vi "SHA-1 Core.vi"(0 "s1":u32=1732584193 format="%.0x", 1 "Input Bytes":u8[](array[numeric]), 5 "s2":u32=4023233417 format="%.0x", 7 "s3":u32=2562383102 format="%.0x", 9 "s4":u32=271733878 format="%.0x", 11 "s5":u32=271733878 format="%.0x") -> (4 "s1 out":u32, 6 "s2 out":u32, 8 "s3 out":u32, 10 "s4 out":u32, 15 "s5 out":u32)   [LabVIEW 2015, in "Front Panel Publisher.lvlib"]
doc: "This VI contains the core of the MD5 algorithm."
uses:
  Front Panel Publisher.lvlib
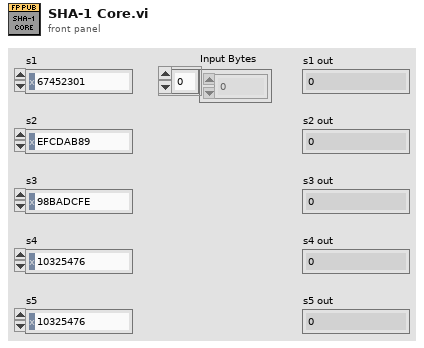
[diagram p1: front panel]
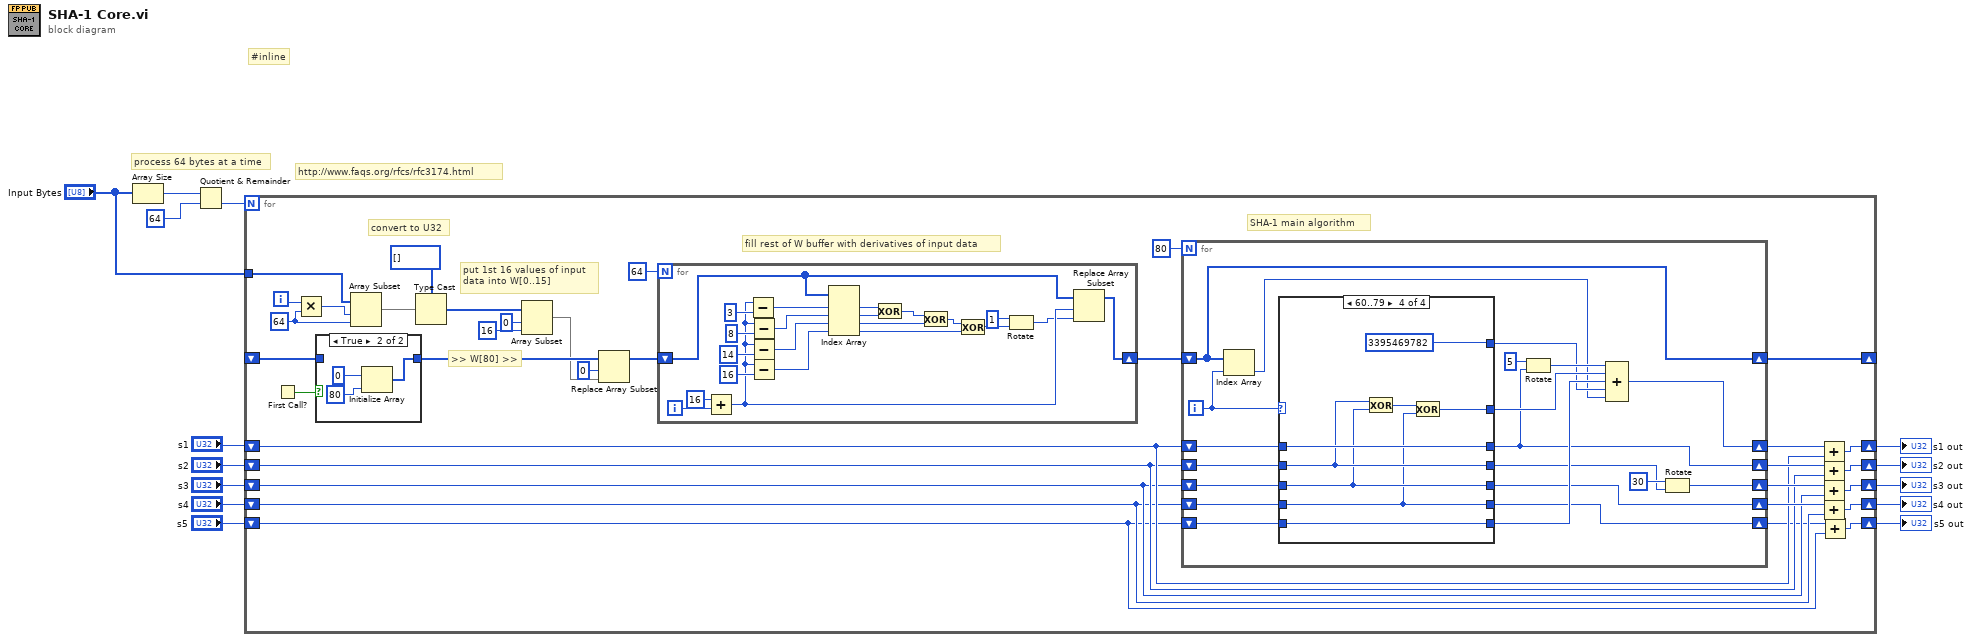
[diagram p0: block diagram]
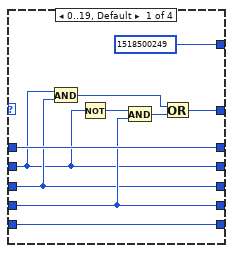
[diagram p2: hidden frame]
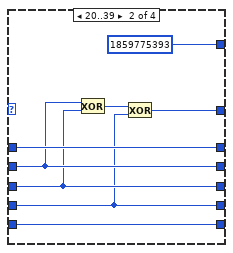
[diagram p3: hidden frame]
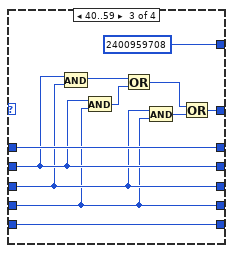
[diagram p4: hidden frame]
diagram:
  # "#inline"
  # "process 64 bytes at a time"
  # "http://www.faqs.org/rfcs/rfc3174.html"
  n1 = Array Size(array="Input Bytes") -> (size(s)=w2:i32)
  n2 = Quotient & Remainder(x=w2, y=64) -> (floor(x/y)=w14:i32)  [unwired: 1 out]
  n3 = for {
    N: w14 -> [_]
    shift-right: [w44] -> w12
    shift-left: "s1" -> [w40]
    shift-right: [w43] -> w11
    shift-left: "s2" -> [w39]
    shift-right: [w42] -> w10
    shift-left: "s3" -> [w38]
    shift-right: [w41] -> w9
    shift-left: "s4" -> [w37]
    tunnel: "Input Bytes" -> [w33]
    shift-right: [w34] -> w3
    shift-left: "s5" -> [w30]
    shift-right: [w19] -> _
    shift-left: _ -> [w24]
    i -> [w36]
    w32 = 64 ("y")
    # "SHA-1 main algorithm"
    # "fill rest of W buffer with derivatives of input data"
    # ">> W[80] >>"
    # "put 1st 16 values of input data into W[0..15]"
    # "convert to U32"
    n4 = First Call?() -> (First Call?: T/F=w26:bool)
    n5 = Multiply(x=w36, y=w32) -> (x*y=w31:i32)
    n6 = case shown="True" w26 {
      tunnel: [w128 w130] -> w25
      tunnel: w24 -> [w128 _]
      frame False {
      }
      frame True {
        n7 = Initialize Array(u32 0 ("y"), 80 ("dimension size")) -> (w130:u32[])
      }
    }
    n8 = Array Subset(array=w33, index=w31, length=w32) -> (w28:u8[])
    n9 = Type Cast(type=u32[] [], x=w28) -> (*(type *) &x=w27:u32[])
    n10 = Array Subset(array=w27, index=0, length=16) -> (w18:u32[])
    n11 = Replace Array Subset(array=w25, new element=w18, index=0) -> (w23:u32[])
    n12 = for {
      N: 64 -> [_]
      shift-right: [w117] -> w20
      shift-left: w23 -> [w115]
      i -> [w127]
      n13 = Add(x=16, y=w127) -> (x+y=w116:i32)
      n14 = Subtract(x=w116, y=3) -> (x-y=w123:i32)
      n15 = Subtract(x=w116, y=8) -> (x-y=w120:i32)
      n16 = Subtract(x=w116, y=14) -> (x-y=w119:i32)
      n17 = Subtract(x=w116, y=16) -> (x-y=w118:i32)
      n18 = Index Array(array=w115, index #1=w123, index #2=w120, index #3=w119, index #4=w118) -> (element #1=w114:u32, element #2=w113:u32, element #3=w111:u32, element #4=w109:u32)
      n19 = Exclusive Or(1:w113, 2:w114) -> (0:w112:u32)
      n20 = Exclusive Or(1:w111, 2:w112) -> (0:w110:u32)
      n21 = Exclusive Or(1:w109, 2:w110) -> (0:w108:u32)
      n22 = Rotate(1:w108, 2:i8 1 ("y")) -> (0:w107:u32)
      n23 = Replace Array Subset(array=w115, new element=w107, index=w116) -> (w117:u32[])
    }
    n24 = for {
      N: 80 -> [_]
      shift-right: [w56] -> w45
      shift-left: w40 -> [w68]
      shift-right: [w55] -> w46
      shift-left: w39 -> [w67]
      shift-right: [w52] -> w47
      shift-left: w38 -> [w66]
      shift-right: [w51] -> w48
      shift-left: w37 -> [w65]
      shift-right: [w50] -> w35
      shift-left: w30 -> [w64]
      shift-right: [w49] -> w19
      shift-left: w20 -> [w49]
      i -> [w58]
      n25 = Index Array(array=w49, index=w58) -> (element=w57:u32)
      n26 = case shown="60..79" w58 {
        tunnel: w68 -> [w73 w86 w97 w104]
        tunnel: w67 -> [w69 w83 w92 w100]
        tunnel: w66 -> [w70 w82 w88 w99]
        tunnel: w65 -> [w72 w80 w87 w98]
        tunnel: w64 -> [w71 w85 w96 w103]
        tunnel: [w73 w86 w97 w104] -> w55
        tunnel: [w69 w83 w92 w100] -> w53
        tunnel: [w70 w82 w88 w99] -> w51
        tunnel: [w72 w80 w87 w98] -> w50
        tunnel: [w71 w85 w96 w103] -> w60
        tunnel: [w75 w79 w89 w101] -> w61
        tunnel: [u32 1518500249 u32 1859775393 u32 2400959708 u32 3395469782] -> w59
        frame 0..19, Default {
          n27 = And(x=w69, y=w70) -> (x .and. y?=w76:u32)
          n28 = Not(x=w69) -> (.not. x?=w78:u32)
          n29 = And(x=w78, y=w72) -> (x .and. y?=w77:u32)
          n30 = Or(x=w76, y=w77) -> (x .or. y?=w75:u32)
        }
        frame 20..39 {
          n31 = Exclusive Or(1:w82, 2:w83) -> (0:w81:u32)
          n32 = Exclusive Or(1:w80, 2:w81) -> (0:w79:u32)
        }
        frame 40..59 {
          n33 = And(x=w92, y=w88) -> (x .and. y?=w93:u32)
          n34 = And(x=w92, y=w87) -> (x .and. y?=w94:u32)
          n35 = Or(x=w93, y=w94) -> (x .or. y?=w91:u32)
          n36 = And(x=w88, y=w87) -> (x .and. y?=w90:u32)
          n37 = Or(x=w91, y=w90) -> (x .or. y?=w89:u32)
        }
        frame 60..79 {
          n38 = Exclusive Or(1:w99, 2:w100) -> (0:w102:u32)
          n39 = Exclusive Or(1:w98, 2:w102) -> (0:w101:u32)
        }
      }
      n40 = Rotate(1:w55, 2:i8 5 ("y")) -> (0:w62:u32)
      n41 = Compound Arithmetic op=ADD(w62, w61, w60, w59, w57) -> (w56:u32)
      n42 = Rotate(1:w53, 2:i8 30 ("y")) -> (0:w52:u32)
    }
    n43 = Add(x=w45, y=w40) -> (x+y=w44:u32)
    n44 = Add(x=w46, y=w39) -> (x+y=w43:u32)
    n45 = Add(x=w47, y=w38) -> (x+y=w42:u32)
    n46 = Add(x=w48, y=w37) -> (x+y=w41:u32)
    n47 = Add(x=w35, y=w30) -> (x+y=w34:u32)
  }
  "s1 out" <- w12
  "s2 out" <- w11
  "s3 out" <- w10
  "s4 out" <- w9
  "s5 out" <- w3
